vi "test2.vi"() -> ()   [LabVIEW 2022 SP3]
panel:
  out "String":string
  in  "Ring":u16(ring) items=["", "Touch Sensor", "Color Sensor"]
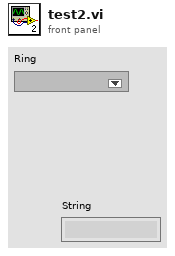
[diagram p1: front panel]
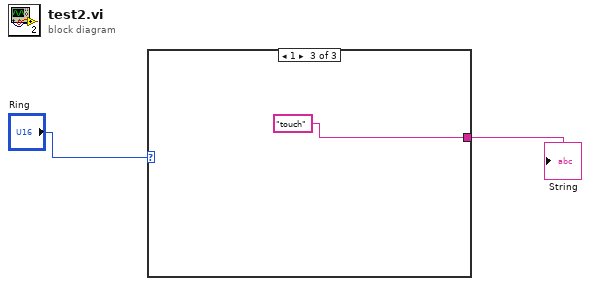
[diagram p0: block diagram]
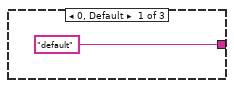
[diagram p2: hidden frame]
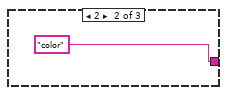
[diagram p3: hidden frame]
diagram:
  n1 = case shown="1" "Ring" {
    tunnel: ["default" "color" "touch"] -> w1
    frame 0, Default {
    }
    frame 2 {
    }
    frame 1 {
    }
  }
  "String" <- w1
